vi "generate_DAC_voltages_V4_justFPGATrajectory.vi"(7 "focus mode?":bool, 8 "derived values":T1, 9 "scan specification":T4={"x amplitude"=0, "x resolution (pixels)"=0, "x offset fly-forward (iterations)"=0, "x offset fly-back (iterations)"=0, "y resolution (nr. of lines)"=0, "y step size"=0, "iterations per pixel"=0, "number of frames"=0, "y offset (pixels)"=0, "number of y-brake lines  (before y-fly-back)"=0, "number y-brake lines (after y-fly-back)"=0, "number of y-fly-back steps"=8, "lines per z step"=0, "number of z/intensity tuples"=0, "number of repetitions (volumes or planes)"=0, "z step size derived"=0, "choose the beginning of z scan"=FALSE, "number of frames (settings)"=0, "FPGA trajectory?"=FALSE, "Pockels cell voltage (bits)"=0, "Vy min(bits)"=0, "Vz min(bits)"=0}, 10 "counter cluster in":T2, 11 "resonant trigger":bool) -> (0 "acquire?":bool, 1 "fly-back acquisition phase?":bool, 2 "counter cluster out":T2, 3 "DAC voltages":T3 {"ch6" max=4095 step=1; "ch5" max=4095 step=1; "ch4" max=4095 step=1; "ch3" max=4095 step=1; "ch2" max=4095 step=1; "ch1" max=4095 step=1; "ch0" max=4095 step=1})   [LabVIEW 2010]
uses:
  scan_specification_cluster.ctl
  common_typedefs/DAC_voltage_cluster.ctl
  counter_cluster.ctl
  derived_values_cluster.ctl
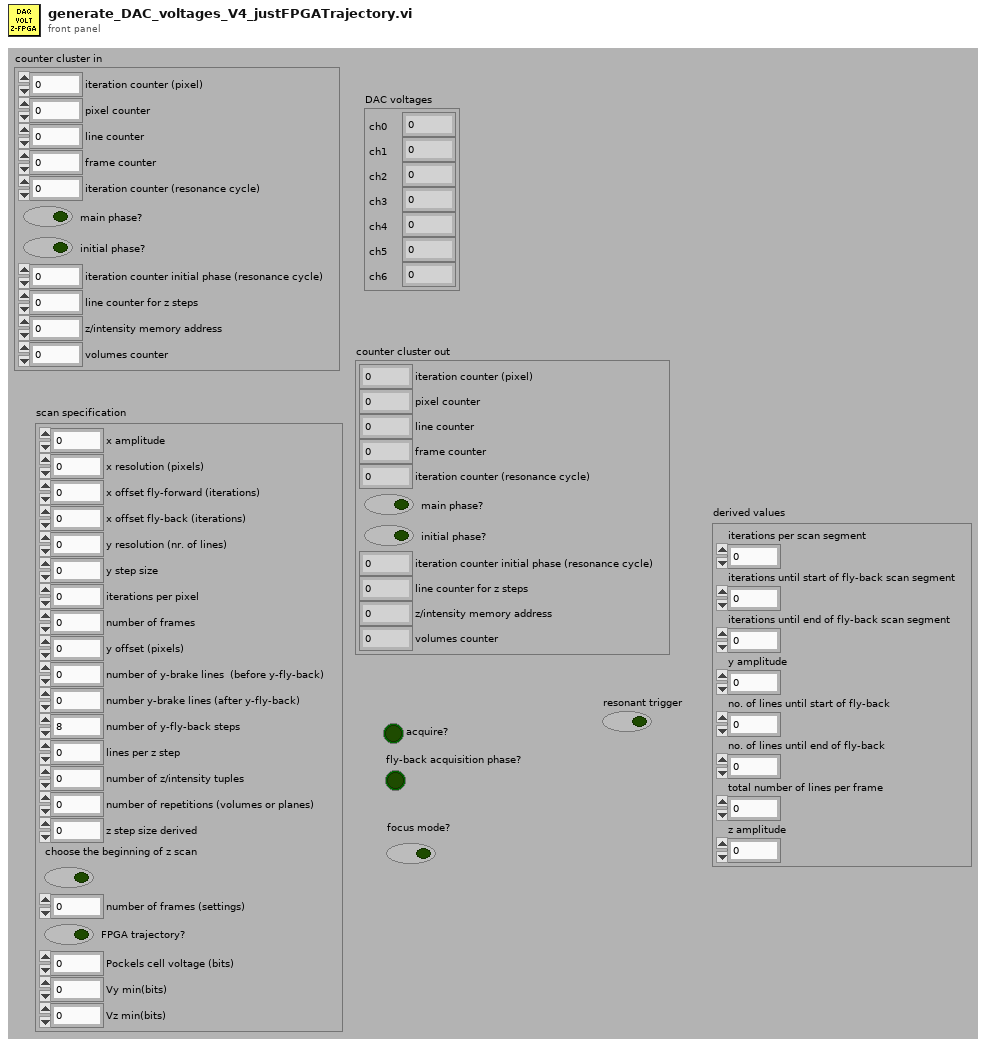
[diagram p1: front panel]
types:
  T1 = typedef "derived_values_cluster.ctl" = cluster{"iterations per scan segment":u16, "iterations until start of fly-back scan segment":u16, "iterations until end of fly-back scan segment":u16, "y amplitude":u16, "no. of lines until start of fly-back":u16, "no. of lines until end of fly-back":u16, "total number of lines per frame ":u16, "z amplitude":u16}
  T2 = typedef "counter_cluster.ctl" = cluster{"iteration counter (pixel)":u16, "pixel counter":u16, "line counter":u16, "frame counter":u16, "iteration counter (resonance cycle)":u16, "main phase?":bool, "initial phase?":bool, "iteration counter initial phase (resonance cycle)":u16, "line counter for z steps":u16, "z/intensity memory address":u32, "volumes counter":u16}
  T3 = typedef "DAC_voltage_cluster.ctl" = cluster{"ch0":u16, "ch1":i16, "ch2":i16, "ch3":i16, "ch4":u16, "ch5":u16, "ch6":u16}
  T4 = typedef "scan_specification_cluster.ctl" = cluster{"x amplitude":u16, "x resolution (pixels)":u16, "x offset fly-forward (iterations)":u16, "x offset fly-back (iterations)":u16, "y resolution (nr. of lines)":u16, "y step size":u16, "iterations per pixel":u16, "number of frames":i32, "y offset (pixels)":u16, "number of y-brake lines  (before y-fly-back)":u16, "number y-brake lines (after y-fly-back)":u16, "number of y-fly-back steps":u16, "lines per z step":u16, "number of z/intensity tuples":u16, "number of repetitions (volumes or planes)":i32, "z step size derived":u16, "choose the beginning of z scan":bool, "number of frames (settings)":i32, "FPGA trajectory?":bool, "Pockels cell voltage (bits)":i16, "Vy min(bits)":i16, "Vz min(bits)":i16}
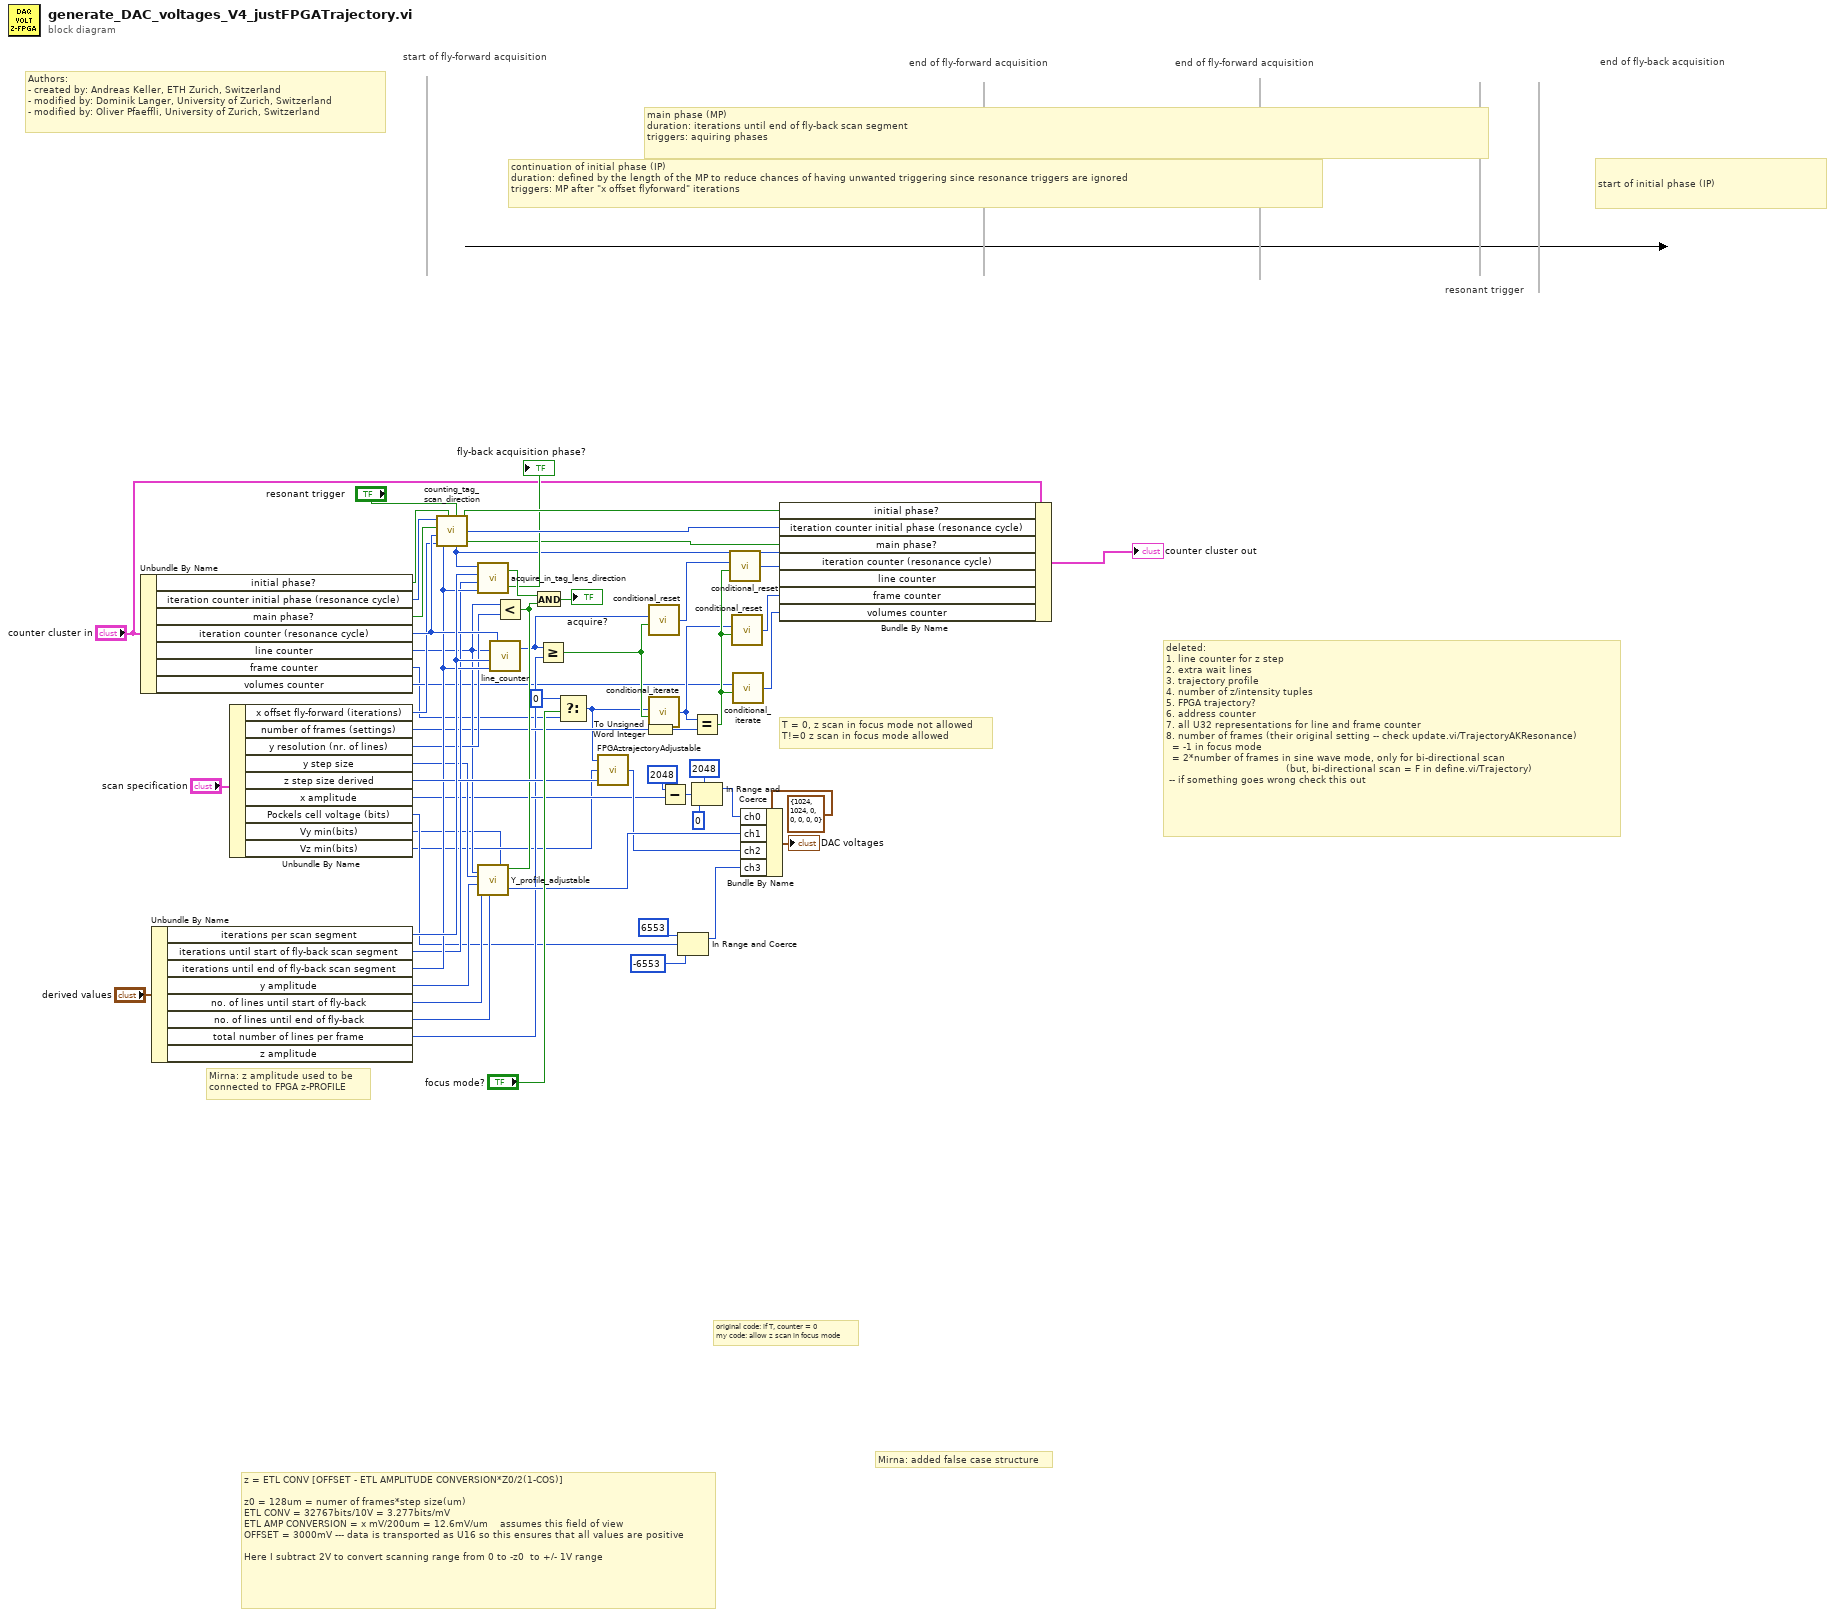
[diagram p0: block diagram]
diagram:
  # "Mirna: z amplitude used to be \nconnected to FPGA z-PROFILE"
  # "T = 0, z scan in focus mode not allowed\nT!=0 z scan in focus mode allowed"
  # "deleted: \n1. line counter for z step\n2. extra wait lines\n3. trajectory profile\n4. number of z/intensity tuples\n5. FPGA trajectory?\n6. address counter\n7. all U32 representations for line and frame counter\n8. number of frames (their original setting -- check update.vi/TrajectoryAKResonance)\n  = -1 in focus mode \n  = 2*number of frames in sine wave mode, only for bi-directional scan\n                                        (but, bi-directional scan = F in define.vi/Trajectory)\n -- if something goes wrong check this out"
  # "z = ETL CONV [OFFSET - ETL AMPLITUDE CONVERSION*Z0/2(1-COS)]\n\nz0 = 128um = numer of frames*step size(um)\nETL CONV = 32767bits/10V = 3.277bits/mV\nETL AMP CONVERSION = x mV/200um = 12.6mV/um    assumes this field of view\nOFFSET = 3000mV --- data is transported as U16 so this ensures that all values are positive\n\nHere I subtract 2V to convert scanning range from 0 to -z0  to +/- 1V range"
  # "original code: if T, counter = 0\nmy code: allow z scan in focus mode"
  # "Mirna: added false case structure"
  # "start of initial phase (IP)"
  # "continuation of initial phase (IP)\nduration: defined by the length of the MP to reduce chances of having unwanted triggering since resonance triggers are ignored\ntriggers: MP after \"x offset flyforward\" iterations"
  # "end of fly-back acquisition"
  # "end of fly-forward acquisition"
  # "end of fly-forward acquisition"
  # "start of fly-forward acquisition"
  # "main phase (MP)\nduration: iterations until end of fly-back scan segment\ntriggers: aquiring phases"
  # "resonant trigger"
  # "Authors: \n- created by: Andreas Keller, ETH Zurich, Switzerland\n- modified by: Dominik Langer, University of Zurich, Switzerland\n- modified by: Oliver Pfaeffli, University of Zurich, Switzerland"
  n1 = Unbundle By Name("counter cluster in") -> ("initial phase?"=w49:bool, "iteration counter initial phase (resonance cycle)"=w36:u16, "main phase?"=w44:bool, "iteration counter (resonance cycle)"=w35:u16, "line counter"=w19:u16, "frame counter"=w9:u16, "volumes counter"=w11:u16)
  n2 = Unbundle By Name("derived values") -> ("iterations per scan segment"=w48:u16, "iterations until start of fly-back scan segment"=w33:u16, "iterations until end of fly-back scan segment"=w34:u16, "y amplitude"=w40:u16, "no. of lines until start of fly-back"=w28:u16, "no. of lines until end of fly-back"=w27:u16, "total number of lines per frame"=w15:u16)  [unwired: 1 out]
  n3 = Unbundle By Name("scan specification") -> ("x offset fly-forward (iterations)"=w31:u16, "number of frames (settings)"=w16:i32, "y resolution (nr. of lines)"=w23:u16, "y step size"=w29:u16, "z step size derived"=w41:u16, "x amplitude"=w17:u16, "Pockels cell voltage (bits)"=w5:i16, "Vy min(bits)"=w2:i16, "Vz min(bits)"=w3:i16)
  n4 = call "counting_tag_scan_direction.vi"("resonant trigger"="resonant trigger", "initial phase?"=w49, "iteration counter initial phase (resonance cycle)"=w36, "main phase?"=w44, "iterations until end of fly-back scan segment"=w34, "iteration counter (resonance cycle)"=w35, "x offset fly-forward (iterations)"=w31) -> ("initial phase? OUT"=w38:bool, "iteration counter initial phase (resonance cycle) out"=w37:u16, "main phase? OUT"=w30:bool, "iteration counter (resonance cycle) out"=w26:u16)
  n5 = call "acquire_in_tag_lens_direction.vi"("iterations until end of fly-back scan segment"=w34, "iterations until start of fly-back scan segment"=w33, "iterations per scan segment"=w48, "iteration counter (resonance cycle) out"=w26) -> ("flyback phase?"=→"fly-back acquisition phase?":bool, "acquire during flyforward or flyback phase?"=w51:bool)
  n6 = call "line_counter.vi"("iterations until end of fly-back scan segment"=w34, "iterations per scan segment"=w48, "line counter in"=w19, "iteration counter (resonance cycle)"=w35) -> ("line counter out"=w14:u16)  [unwired: 1 out]
  n7 = Less?(x=w19, y=w23) -> (x < y?=w22:bool)
  n8 = call "Y_profile_adjustable.vi"("Vy min(bits)"=w2, "no. of lines until end of fly-back"=w27, "line counter"=w19, "no. of lines until start of fly-back"=w28, "y amplitude"=w40, "y step size"=w29, "y acquire? (line counter<number of lines)"=w22) -> ("y signal"=w43:i16)
  n9 = And(x=w51, y=w22) -> (x .and. y?=→"acquire?":bool)
  n10 = Greater Or Equal?(x=w14, y=w15) -> (x >= y?=w18:bool)
  n11 = Select(t=u16 0, s="focus mode?", f=w9) -> (s? t:f=w4:u16)
  n12 = call "FPGAztrajectoryAdjustable.vi"("z step size derived"=w41, "Vz min (bits)"=w3, "z/intensity memory address"=w4) -> ("Z trajectory"=w42:i16)
  n13 = To Unsigned Word Integer(number=w16) -> (unsigned 16bit integer=w12:u16)
  n14 = call "conditional_reset.vi"("reset?"=w18, "number in"=w14) -> ("number out"=w24:u16)  [unwired: 4 in]
  n15 = call "conditional_iterate.vi"("iterate?"=w18, "number in"=w4) -> ("number out"=w13:u16)  [unwired: 4 in]
  n16 = Subtract(x=u16 2048, y=w17) -> (x-y=w55:u16)
  n17 = In Range and Coerce(upper limit=i16 6553, x=w5, lower limit=i16 -6553) -> (coerced(x)=w6:i16)  [unwired: 1 out]
  n18 = Equal?(x=w13, y=w12) -> (x = y?=w25:bool)
  n19 = In Range and Coerce(upper limit=u16 2048, x=w55, lower limit=u16 0) -> (coerced(x)=w54:u16)  [unwired: 1 out]
  n20 = call "conditional_reset.vi"("reset?"=w25, "number in"=w24) -> ("number out"=w46:u16)  [unwired: 4 in]
  n21 = call "conditional_reset.vi"("reset?"=w25, "number in"=w13) -> ("number out"=w21:u16)  [unwired: 4 in]
  n22 = call "conditional_iterate.vi"("iterate?"=w25, "number in"=w11) -> ("number out"=w47:u16)  [unwired: 4 in]
  n23 = Bundle By Name(cluster=T3 {"ch0"=1024, "ch1"=1024, "ch2"=0, "ch3"=0, "ch4"=0, "ch5"=0, "ch6"=0} ("DAC voltage"), "ch0"=w54, "ch1"=w43, "ch2"=w42, "ch3"=w6) -> (→"DAC voltages":T3)
  n24 = Bundle By Name(cluster="counter cluster in", "initial phase?"=w38, "iteration counter initial phase (resonance cycle)"=w37, "main phase?"=w30, "iteration counter (resonance cycle)"=w26, "line counter"=w46, "frame counter"=w21, "volumes counter"=w47) -> (→"counter cluster out":T2)
